vi "util-varient-proc-running.vi"(8 "error in":errorcluster, 10 "Enum":enum16{"START", "STOP"}(ring), 11 "Procedure in":variant) -> (0 "error out":errorcluster, 3 "Procedure out":variant)   [LabVIEW 2024]
uses:
  controls/typeProcVarientName.ctl
  Polymorphics/variantCtrlBoolean.vi
  proc.util.validateParamExist.vi
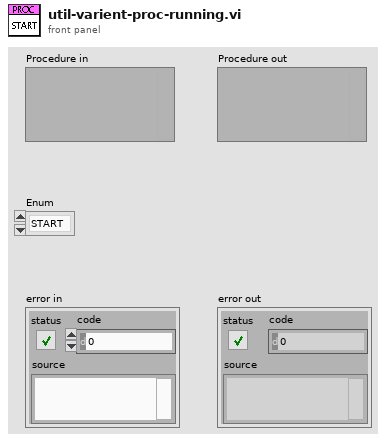
[diagram p1: front panel]
types:
  T1 = typedef "typeProcVarientName.ctl" = enum16{"procNameID", "procModuleID", "procPath", "procIsRunning", "procIndex", "procModule", "procRegisterNumeric", "procRegisterString", "procReport", "procReportPrev", "procCLK", "procStepPointer", "procType"}
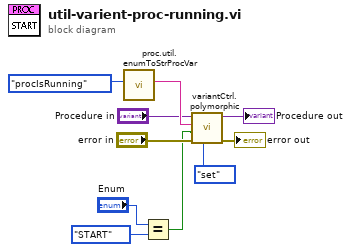
[diagram p0: block diagram]
diagram:
  n1 = call "proc.util.enumToStrProcVar.vi"("Proc var"=typeProcVarientName."procIsRunning" ("Combo Box")) -> ("String"=w7:string)  [unwired: 10 in]
  n2 = Equal?(x="Enum", y=enum16{"START", "STOP"}."START") -> (x = y?=w1:bool)
  n3 = call-poly "variantCtrl.polymorphic.vi"("menu in (get)"=enum16{"get", "set"}."set", "error in"="error in", "Boolean Value in"=w1, "name in"=w7, "variant in"="Procedure in") -> ("error out"=→"error out":errorcluster, "variant out"=→"Procedure out":variant)  [unwired: 3 in, 2 out]
